vi "PH_SHS_Analysis.open or close Zernike Service.vi"(0 "i ref in":refnum<vi>, 2 "open":bool, 5 "error in (no error)":errorcluster) -> (14 "i ref out":refnum<vi>, 19 "error out":errorcluster)   [LabVIEW 2014, in "PH_SHS_Analysis.lvlib"]
doc: "This VI opens (true) or closes (false) the DIM-Service \"<Instance>_Zernikes\"."
uses:
  PH_SHS_Analysis.lvlib
  PH_SHS_Analysis.Zernike Dataset.ctl
  PH_Basics/PH_StatusHandler/PH_StatusHandler.Status.ctl
  PH_SHS_Analysis.Zernike Coefficients.ctl
  PH_Basics/PH_Common/PH_Common.lvlib
  CSlibraries-extern/DimLVEvent/LVDimInterface/LVDimInterface.lvlib
  PH_Basics/PH_StatusHandler/PH_StatusHandler.lvlib
panel:
  in  "SHS Zernicke Dataset":T1 {"State" items=["no info", "off/false/out", "on/true/in", "Failure", "Alarm", "Status 1", "Status 2", "Status 3"]; "Zernicke Coefficients"."2nd Spherical" scale=-2.0..2.0 scale format="%.2f"; "Zernicke Coefficients"."2nd Coma y" scale=-2.0..2.0 scale format="%.2f"; "Zernicke Coefficients"."2nd Coma x" scale=-2.0..2.0 scale format="%.2f"; "Zernicke Coefficients"."2nd Astig 45°" scale=-2.0..2.0 scale format="%.2f"; "Zernicke Coefficients"."2nd Astig 0°" scale=-2.0..2.0 scale format="%.2f"; "Zernicke Coefficients"."Trefoil 30°" scale=-2.0..2.0 scale format="%.2f"; "Zernicke Coefficients"."Trefoil 0°" scale=-2.0..2.0 scale format="%.2f"; "Zernicke Coefficients"."Spherical" scale=-2.0..2.0 scale format="%.2f"; "Zernicke Coefficients"."Coma y" scale=-2.0..2.0 scale format="%.2f"; "Zernicke Coefficients"."Coma x" scale=-2.0..2.0 scale format="%.2f"; "Zernicke Coefficients"."Astig 45°" scale=-2.0..2.0 scale format="%.2f"; "Zernicke Coefficients"."Astig 0°" scale=-2.0..2.0 scale format="%.2f"; "Zernicke Coefficients"."Defocus" scale=-2.0..2.0 scale format="%.2f"; "Zernicke Coefficients"."Tilt y" scale=-2.0..2.0 scale format="%.2f"; "Zernicke Coefficients"."Tilt x" scale=-2.0..2.0 scale format="%.2f"}
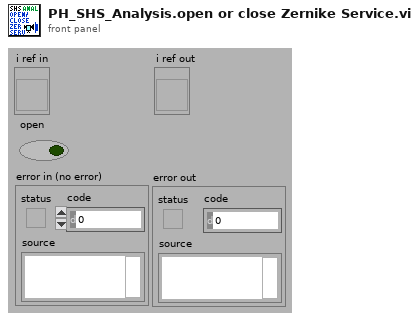
[diagram p1: front panel]
types:
  T1 = typedef "PH_SHS_Analysis.lvlib/PH_SHS_Analysis.Zernike Dataset.ctl" = cluster{"State":T2, "Time Stamp":timestamp, "PtV [lambda]":dbl, "Zernicke Coefficients":T3}
  T2 = typedef "PH_StatusHandler.lvlib/PH_StatusHandler.Status.ctl" = i16
  T3 = typedef "PH_SHS_Analysis.lvlib/PH_SHS_Analysis.Zernike Coefficients.ctl" = cluster{"Tilt x":dbl, "Tilt y":dbl, "Defocus":dbl, "Astig 0°":dbl, "Astig 45°":dbl, "Coma x":dbl, "Coma y":dbl, "Spherical":dbl, "Trefoil 0°":dbl, "Trefoil 30°":dbl, "2nd Astig 0°":dbl, "2nd Astig 45°":dbl, "2nd Coma x":dbl, "2nd Coma y":dbl, "2nd Spherical":dbl}
  T4 = typedef "PH_SHS_Analysis.lvlib/PH_SHS_Analysis.i attribute.ctl" = cluster{"GUI Refs":cluster{"Delete":refnum<vi>, "Global On":refnum<vi>, "Cam Source":refnum<vi>, "Calibration Data File":refnum<vi>, "Calibration status":refnum<vi>, "Show overlay":refnum<vi>, "SHS Device Config":refnum<vi>, "Result":refnum<vi>, "Consider Tilt":refnum<vi>, "Working Reference":refnum<vi>, "Remove Tilt":refnum<vi>, "Take Cali  Reference":refnum<vi>, "Publishing Data Status":refnum<vi>, "Calibration Data":refnum<vi>}, "Calibration":cluster{"Status":T2, "Data":T5, "File":path}, "Result":T10, "Image":T12, "SHS Device Config":T13, "Show Overlay":bool, "GradientZernikeMatrix":dbl[][], "Consider Tilt":bool, "Working Reference":T6, "Zernicke Service ID":i32, "PSDB Image":T12}
  T5 = typedef "PH_SHS_Analysis_Calibrator.lvlib/PH_SHS_Analysis_Calibrator.Analysis Calibration Data.ctl" = cluster{"Date":string, "Time":string, "Cam Settings":cluster{"Cam ID":string, "Gain":dbl, "Brightness":dbl, "Shutter":dbl, "Cam Error":bool, "Mode":i32}, "SHS Reference Result":T6, "Pixel Size":dbl, "MLA Pitch":dbl, "Method":enum16{"automatic", "manual"}, "Calibration Data calculated":bool, "No Problems at calculation?":bool, "error out":errorcluster}
  T6 = typedef "SHS_Common.lvlib/SHSReference.ctl" = cluster{"Reference":T7[][], "Lens Array Pitch [px]":dbl}
  T7 = typedef "SHS_Common.lvlib/ReferencePoint.ctl" = cluster{"Rect":T8, "Point":T9}
  T8 = typedef "SHS_Common.lvlib/Rectangle.ctl" = cluster{"Left":i32, "Top":i32, "Right":i32, "Bottom":i32}
  T9 = typedef "SHS_Common.lvlib/Point.ctl" = cluster{"x":dbl, "y":dbl, "valid?":bool, "weight":dbl}
  T10 = typedef "PH_SHS_Analysis.lvlib/PH_SHS_Analysis.Result.ctl" = cluster{"Time Stamp":timestamp, "Zernike Coefficients":T3, "PtV [lambda]":dbl, "Shifts":T11, "Measurement Quality":cluster{dbl, dbl, dbl}, "Measurement valid?":bool}
  T11 = typedef "SHS_Common.lvlib/Shifts.ctl" = T9[][]
  T12 = typedef "IMAQ Image.ctl" = refnum<image>
  T13 = typedef "SHS_Analysis.lvlib/SHS_DeviceConfig.ctl" = cluster{"focal length [m]":dbl, "pixel size [m/px]":dbl, "wavelength [m]":dbl}
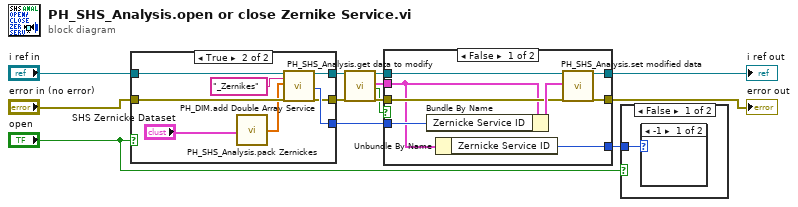
[diagram p0: block diagram]
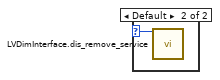
[diagram p2: hidden frame]
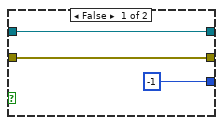
[diagram p4: hidden frame]
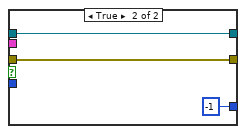
[diagram p5: hidden frame]
diagram:
  n1 = case shown="True" "open" {
    tunnel: "error in (no error)" -> [w14 w24]
    tunnel: "i ref in" -> [w15 w23]
    tunnel: [-1 ("Service ID") w22] -> w9
    tunnel: [w15 w19] -> w8
    tunnel: [w14 w18] -> w6
    frame False {
    }
    frame True {
      n2 = call "PH_SHS_Analysis.pack Zernickes.vi"("SHS Zernicke Dataset"="SHS Zernicke Dataset") -> ("DIM Service Array"=w21:dbl[])
      n3 = call "PH_DIM.add Double Array Service.vi"("i ref in"=w23, "Service Name"="_Zernikes", "Double Value Array"=w21, "error in (no error)"=w24) -> ("i ref out"=w19:refnum<vi>, "Service ID"=w22:i32, "error out"=w18:errorcluster)  [unwired: 13 in]
    }
  }
  n4 = call "PH_SHS_Analysis.get data to modify.vi"("i ref in"=w8, "error in (no error)"=w6) -> ("i ref out"=w7:refnum<vi>, "i attribute"=w4:T4, "timed out"=w3:bool, "error out"=w5:errorcluster)  [unwired: 14 in]
  n5 = case shown="False" w3 {
    tunnel: [w32 w35] -> w12
    tunnel: [w31 w34] -> w13
    tunnel: w9 -> [w29 _]
    tunnel: w7 -> [w28 w35]
    tunnel: w5 -> [w27 w34]
    tunnel: w4 -> [w26 _]
    tunnel: [w25 -1 ("Zernicke Service ID")] -> w2
    frame False {
      n6 = Bundle By Name(cluster=w26, "Zernicke Service ID"=w29) -> (w30:T4)
      n7 = Unbundle By Name(w26) -> ("Zernicke Service ID"=w25:i32)
      n8 = call "PH_SHS_Analysis.set modified data.vi"("i ref in"=w28, "i attribute"=w30, "error in (no error)"=w27) -> ("i ref out"=w32:refnum<vi>, "error out"=w31:errorcluster)  [unwired: 15 in]
    }
    frame True {
    }
  }
  "error out" <- w13
  "i ref out" <- w12
  n9 = case shown="False" "open" {
    tunnel: w2 -> [w36 _]
    frame False {
      n10 = case shown="-1" w36 {
        selector: w36 -> [_ w37]
        frame -1 {
        }
        frame Default {
          n11 = call "LVDimInterface.dis_remove_service.vi"("my_serviceID"=w37) -> ()  [unwired: 18 in, 1 out]
        }
      }
    }
    frame True {
    }
  }
